vi "DateString.vi"() -> (1 "full date string":string, 2 "date string":string, 3 "time string":string, 4 "Year":string, 6 "Month":string)   [LabVIEW 2018]
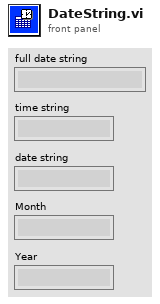
[diagram p1: front panel]
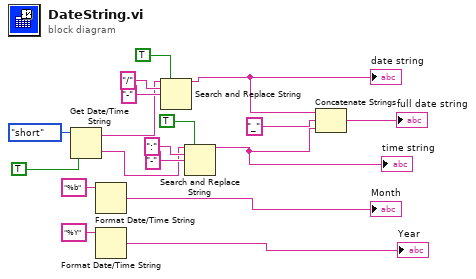
[diagram p0: block diagram]
diagram:
  n1 = Get Date/Time String(date format (0)=enum16{"short", "long", "abbreviated"}."short", want seconds? (F)=TRUE) -> (date string=w16:string, time string=w1:string)  [unwired: 1 in]
  n2 = Format Date/Time String(time format string (%c)="%b") -> (date/time string=→"Month":string)  [unwired: 2 in]
  n3 = Format Date/Time String(time format string (%c)="%Y") -> (date/time string=→"Year":string)  [unwired: 2 in]
  n4 = Search and Replace String(replace all?=TRUE ("replace all? (F)"), input string=w16, search string="/", replace string="-" ("replace string (\"\")")) -> (result string=w12:string)  [unwired: 4 in, 3 out]
  "date string" <- w12
  n5 = Search and Replace String(replace all?=TRUE ("replace all? (F)"), input string=w1, search string=":", replace string="-" ("replace string (\"\")")) -> (result string=w2:string)  [unwired: 4 in, 3 out]
  "time string" <- w2
  n6 = Concatenate Strings(w12, "_", w2) -> (→"full date string":string)
